vi "Shock.vi"() -> ()   [LabVIEW 2012]
uses:
  <vilib>/Instr/_visa.llb/Select Event Type.ctl
  <instrlib>/niHWS/nihws.llb/niHWS Open File Permissions ID.ctl
  <vilib>/DAQmx/write.llb/DAQmx Write (Digital Bool 1Line 1Point).vi
  <instrlib>/niHWS/nihws.llb/niHWS Write Analog WDT.vi
  <vilib>/DAQmx/miscellaneous.llb/DAQmx Fill In Error Info.vi
  <vilib>/express/express arith-compare/Formula/XNode/ExpressFormulaBlockNode.xnode
  <vilib>/ptbypt/NI_PtbyPt.lvlib
panel:
  out "Shock Countdown":dbl
  in  "Random":bool
  in  "shock time (ms)":u32
  in  "Shock Button":bool
  out "Shock":bool
  out "Click Value":i8
  out "Speed History":dbl(graph)
  in  "stop":bool
  out "Rec Time":dbl format="%#_3g"
  in  "Rec":bool
  in  "Path":path
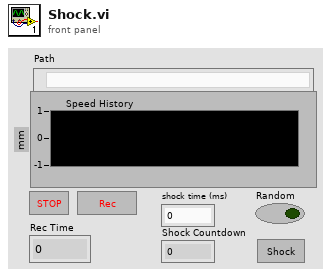
[diagram p1: front panel]
types:
  T1 = typedef "niHWS Open File Permissions ID.ctl" = enum32{"Read Only", "Read/Write Existing", "Read/Write/Create New", "Read/Write/Create New Always"}
  T2 = typedef "Select Event Type.ctl" = u32
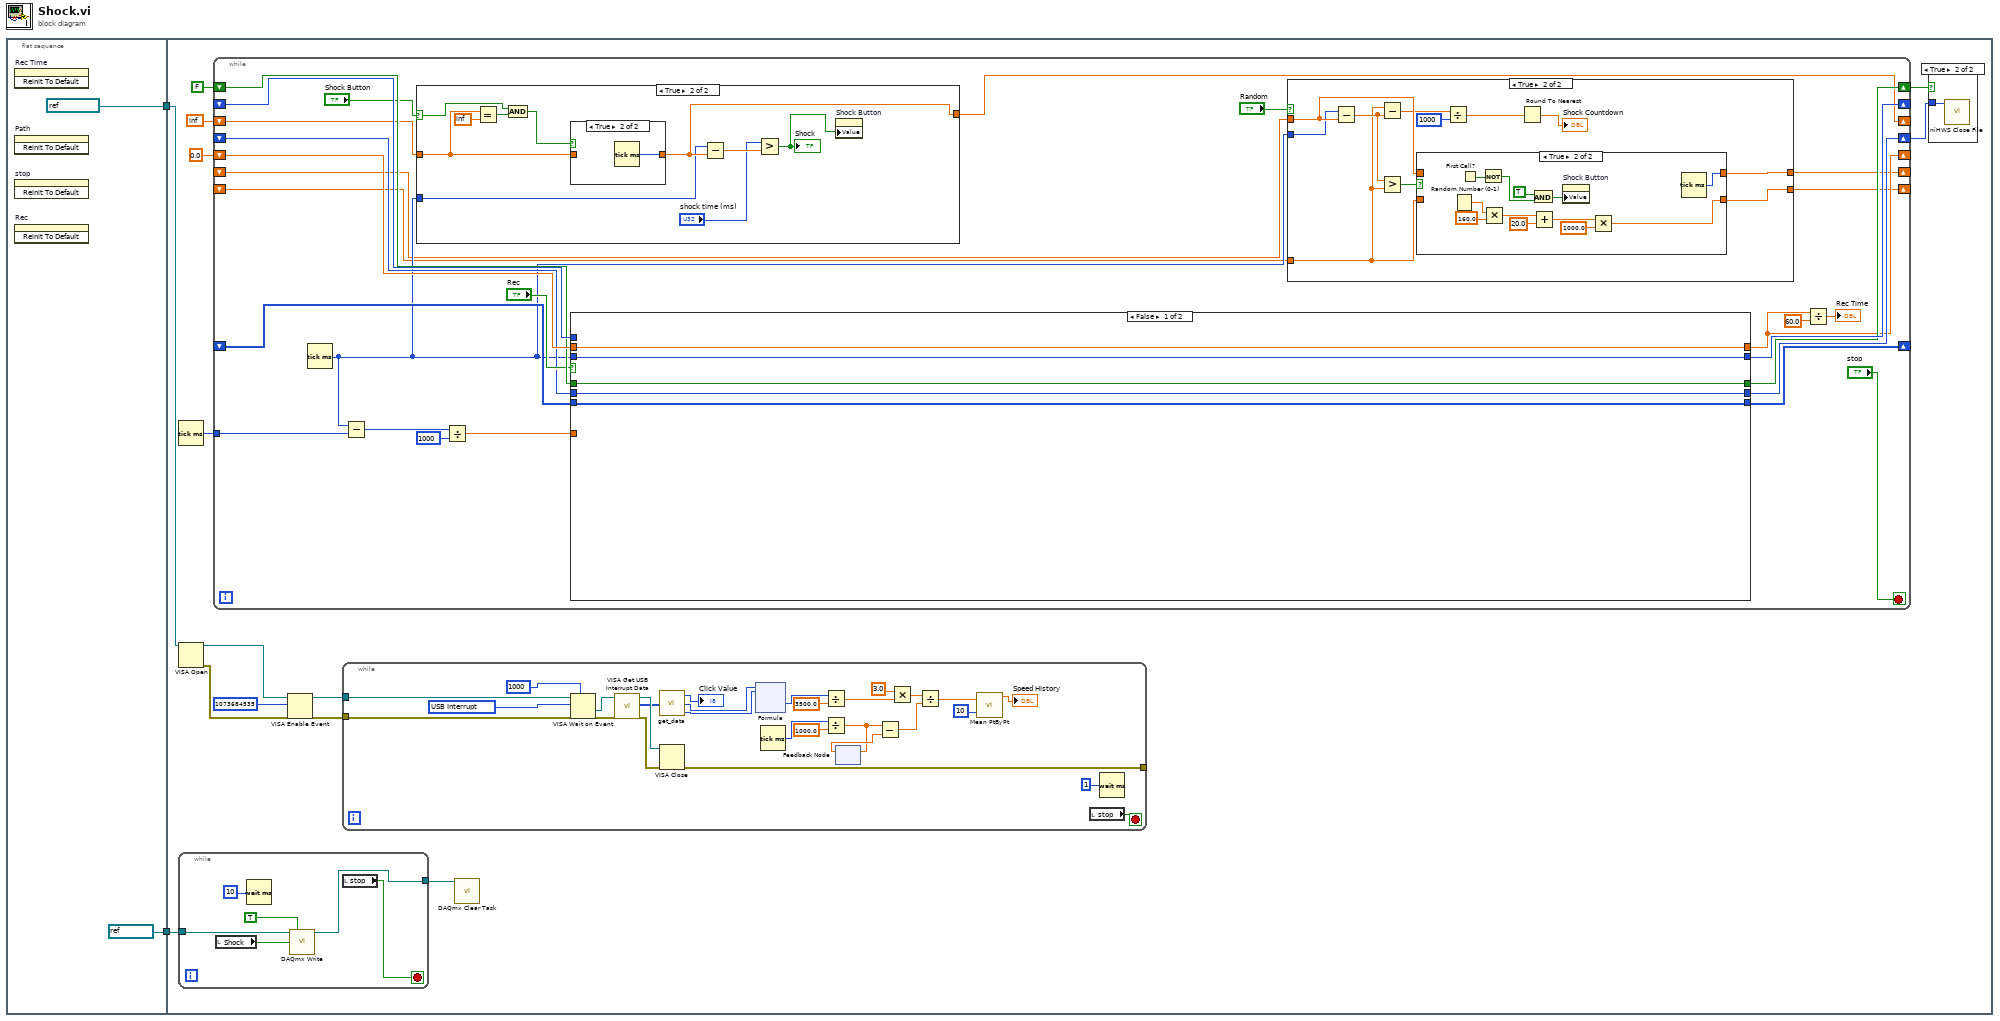
[diagram p0: block diagram]
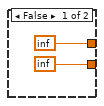
[diagram p3: hidden frame]
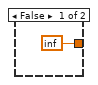
[diagram p5: hidden frame]
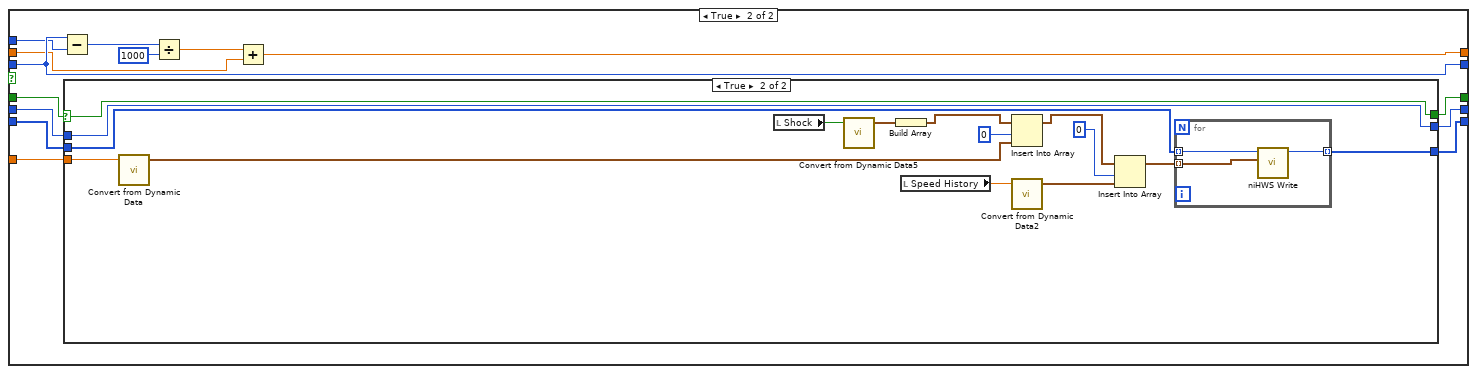
[diagram p7: hidden frame]
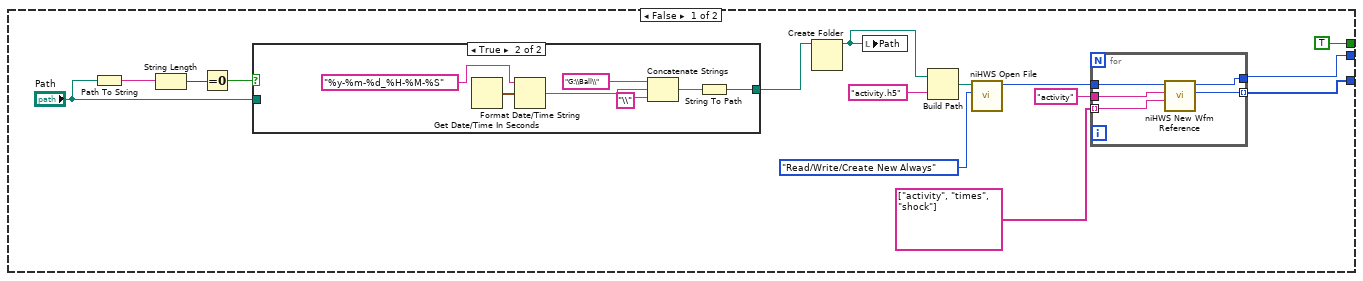
[diagram p8: hidden frame]
diagram:
  n1 = flat-sequence {
    tunnel: [refnum<visa-resource-name> "Mouse2" ("VISA resource name")] -> w2
    tunnel: [refnum<k21> "Shock" ("task/channels in")] -> w1
    tunnel: w2 -> [w8]
    tunnel: w1 -> [w7]
    frame #0 {
      n2 = invoke on="Rec Time" class="DigNum (strict)" method="Reinit To Default"() -> ()  [unwired: 3 in, 3 out]
      n3 = invoke on="Path" class="Path" method="Reinit To Default"() -> ()  [unwired: 3 in, 3 out]
      n4 = invoke on="stop" class="Bool (strict)" method="Reinit To Default"() -> ()  [unwired: 3 in, 3 out]
      n5 = invoke on="Rec" class="Bool (strict)" method="Reinit To Default"() -> ()  [unwired: 3 in, 3 out]
    }
    frame #1 {
      n6 = Tick Count (ms)() -> (millisecond timer value=w17:u32)
      n7 = VISA Open(VISA resource name=w8) -> (VISA resource name=w11:refnum<visa-resource-name>, error out=w10:errorcluster)  [unwired: 1 in, 3 out]
      n8 = while {
        tunnel: w7 -> [w60]
        tunnel: [w59] -> w6
        stop <- w62 stop-if-true
        n9 = local read "Shock"() -> (w57:bool)
        n10 = Wait (ms)(milliseconds to wait=u32 10) -> ()  [unwired: 1 out]
        n11 = call-poly <vilib>:"DAQmx Write.vi"("task/channels in"=w60, "auto start"=TRUE, "data"=w57) -> ("task out"=w59:refnum<k21>)  [unwired: 10 in, 2 out]
        n12 = local read "stop"() -> (w62:bool)
      }
      n13 = while {
        tunnel: w17 -> [w90]
        shift-right: [w89] -> _
        shift-left: _ -> [w88]
        shift-right: [w75] -> _
        shift-left: 0.0 -> [w87]
        shift-right: [w81] -> w15
        shift-left: FALSE -> [w82]
        shift-right: [w78] -> _
        shift-left: _ -> [w77]
        shift-right: [w79] -> w14
        shift-left: _ -> [w76]
        shift-right: [w71] -> _
        shift-left: inf -> [w70]
        shift-right: [w68] -> _
        shift-left: _ -> [w66]
        shift-right: [w65] -> _
        shift-left: _ -> [w64]
        stop <- "stop" stop-if-true
        n14 = Tick Count (ms)() -> (millisecond timer value=w67:u32)
        n15 = Subtract(x=w67, y=w90) -> (x-y=w85:u32)
        n16 = case shown="True" "Shock Button" {
          selector: "Shock Button" -> [_ w121]
          tunnel: w67 -> [_ w127]
          tunnel: [inf w128] -> w71
          tunnel: w70 -> [_ w123]
          frame False {
          }
          frame True {
            n17 = Equal?(x=w123, y=inf) -> (x = y?=w122:bool)
            n18 = And(x=w121, y=w122) -> (x .and. y?=w120:bool)
            n19 = case shown="True" w120 {
              tunnel: [w129 w130] -> w128
              tunnel: w123 -> [w129 _]
              frame False {
              }
              frame True {
                n20 = Tick Count (ms)() -> (millisecond timer value=w130:u32)
              }
            }
            n21 = Subtract(x=w127, y=w128) -> (x-y=w126:dbl)
            n22 = Greater?(x="shock time (ms)", y=w126) -> (0:w119:bool)
            "Shock" <- w119
            n23 = property on="Shock Button" class="Bool (strict)"("Value"=w119) -> ()  [unwired: 2 in, 2 out]
          }
        }
        n24 = Divide(x=w85, y=1000) -> (x/y=w83:dbl)
        n25 = case shown="False" "Rec" {
          tunnel: [w134 w146] -> w75
          tunnel: w83 -> [_ w140]
          tunnel: [w135 w149] -> w89
          tunnel: w67 -> [w135 w149]
          tunnel: w88 -> [_ w148]
          tunnel: w87 -> [w134 w147]
          tunnel: w82 -> [w133 w142]
          tunnel: [w133 w141] -> w81
          tunnel: [w131 w139] -> w79
          tunnel: [w132 w138] -> w78
          tunnel: w77 -> [w132 w137]
          tunnel: w76 -> [w131 w136]
          frame False {
          }
          frame True {
            n26 = Subtract(x=w149, y=w148) -> (x-y=w145:u32)
            n27 = case shown="True" w142 {
              selector: w142 -> [_ w192]
              tunnel: [TRUE w192] -> w141
              tunnel: w140 -> [_ w189]
              tunnel: [w152 w191] -> w139
              tunnel: [w151 w181] -> w138
              tunnel: w137 -> [_ w182]
              tunnel: w136 -> [_ w191]
              frame False {
                n28 = Path To String(path="Path") -> (string=w162:string)
                n29 = String Length(string=w162) -> (length=w163:i32)
                n30 = Equal To 0?(x=w163) -> (x = 0?=w158:bool)
                n31 = case shown="True" w158 {
                  tunnel: [w170 w171] -> w156
                  tunnel: "Path" -> [w170 _]
                  frame False {
                  }
                  frame True {
                    n32 = Get Date/Time In Seconds() -> (seconds since 1Jan1904=w177:timestamp)
                    n33 = Format Date/Time String(time format string (%c)="%y-%m-%d_%H-%M-%S", seconds (now)=w177) -> (date/time string=w174:string)  [unwired: 1 in]
                    n34 = Concatenate Strings("G:\\Ball\\", w174, "\\" ("string")) -> (w172:string)
                    n35 = String To Path(string=w172) -> (path=w171:path)
                  }
                }
                n36 = Create Folder(path (use dialog)=w156) -> (created path=w155:path)  [unwired: 2 in, 2 out]
                n37 = local write "Path"(w155) -> ()
                n38 = Build Path(base path=w155, name or relative path="activity.h5" ("search string")) -> (appended path=w159:path)
                n39 = call <instrlib>:"niHWS Open File.vi"("permissions (0:read only)"=niHWS_Open_File_Permissions_ID."Read/Write/Create New Always", "file path"=w159) -> ("file handle"=w150:u32)  [unwired: 8 in, 1 out]
                n40 = for {
                  tunnel: w150 -> [w169]
                  tunnel: [w168] -> w151 mode=indexing
                  tunnel: "activity" ("group name (empty)") -> [w167]
                  tunnel: string[] ["activity", "times", "shock"] -> [w166] mode=indexing
                  tunnel: [w165] -> w152
                  n41 = call <instrlib>:"niHWS New Wfm Reference.vi"("waveform name (empty)"=w166, "group name (empty)"=w167, "file handle in"=w169) -> ("waveform reference"=w168:u32, "file handle out"=w165:u32)  [unwired: 6 in, 1 out]
                }
              }
              frame True {
                n42 = call "Convert from Dynamic Data"("Dynamic Data Type"=w189) -> ("Waveform"=w188:waveform(dbl))  [unwired: 3 in]
                n43 = local read "Shock"() -> (w179:bool)
                n44 = call "Convert from Dynamic Data5"("Dynamic Data Type"=w179) -> ("Waveform"=w180:waveform(dbl))  [unwired: 3 in]
                n45 = Build Array(w180) -> (w178:waveform(dbl)[])
                n46 = local read "Speed History"() -> (w185:dbl)
                n47 = Insert Into Array(array=w178, index=0, new element=w188) -> (w186:waveform(dbl)[])
                n48 = call "Convert from Dynamic Data2"("Dynamic Data Type"=w185) -> ("Waveform"=w184:waveform(dbl))  [unwired: 3 in]
                n49 = Insert Into Array(array=w186, index=0, new element=w184) -> (w183:waveform(dbl)[])
                n50 = for {
                  tunnel: w182 -> [w195] mode=indexing
                  tunnel: w183 -> [w194] mode=indexing
                  tunnel: [w193] -> w181 mode=indexing
                  n51 = call-poly <instrlib>:"niHWS Write.vi"("analog waveform"=w194, "waveform reference in"=w195) -> ("waveform reference out"=w193:u32)  [unwired: 8 in, 1 out]
                }
              }
            }
            n52 = Divide(x=w145, y=1000) -> (x/y=w143:dbl)
            n53 = Add(x=w143, y=w147) -> (x+y=w146:dbl)
          }
        }
        n54 = case shown="True" "Random" {
          tunnel: [inf w103] -> w68
          tunnel: w67 -> [_ w101]
          tunnel: w66 -> [_ w102]
          tunnel: [inf w99] -> w65
          tunnel: w64 -> [_ w97]
          frame False {
          }
          frame True {
            n55 = Subtract(x=w101, y=w102) -> (x-y=w98:dbl)
            n56 = Subtract(x=w97, y=w98) -> (x-y=w96:dbl)
            n57 = Greater?(x=w98, y=w97) -> (0:w100:bool)
            n58 = case shown="True" w100 {
              tunnel: [w105 w113] -> w103
              tunnel: [w104 w111] -> w99
              tunnel: w102 -> [w105 _]
              tunnel: w97 -> [w104 _]
              frame False {
              }
              frame True {
                n59 = Random Number (0-1)() -> (number: 0 to 1=w117:dbl)
                n60 = First Call?() -> (First Call?: T/F=w110:bool)
                n61 = Not(x=w110) -> (.not. x?=w108:bool)
                n62 = Multiply(x=w117, y=160.0) -> (x*y=w114:dbl)
                n63 = And(x=TRUE ("Shock Button"), y=w108) -> (x .and. y?=w107:bool)
                n64 = Add(x=w114, y=20.0) -> (x+y=w112:dbl)
                n65 = property on="Shock Button" class="Bool (strict)"("Value"=w107) -> ()  [unwired: 2 in, 2 out]
                n66 = Multiply(x=w112, y=1000.0) -> (x*y=w111:dbl)
                n67 = Tick Count (ms)() -> (millisecond timer value=w113:u32)
              }
            }
            n68 = Divide(x=w96, y=1000) -> (x/y=w95:dbl)
            n69 = Round To Nearest(number=w95) -> (nearest integer value=→"Shock Countdown":dbl)
          }
        }
        n70 = Divide(x=w75, y=60.0) -> (x/y=→"Rec Time":dbl)
      }
      n71 = VISA Enable Event(8:w10, 10:u32 1073684535 ("event type"), 11:w11) -> (0:w13:errorcluster, 3:w12:refnum<visa-resource-name>)  [unwired: 1 out]
      n72 = while {
        tunnel: w12 -> [w46]
        tunnel: [w45] -> _
        tunnel: w13 -> [w38]
        stop <- w39 stop-if-true
        w37 = T2 1073684535 items=["Service Request"=1073684491, "Trigger"=3221168138, "Clear"=1073684493, "VXI Signal"=1073684512, "VXI/VME Interrupt"=3221168161, "VXI/VME Sysfail"=1073684509, "VXI/VME Sysreset"=1073684510, "GPIB CIC"=1073684498, "GPIB Talk"=1073684499, "GPIB Listen"=1073684500, "PXI Interrupt"=1073684514, "Serial Break"=1073684515, "Serial TermChar"=1073684516, "Serial CTS"=1073684521, "Serial DSR"=1073684522, "Serial DCD"=1073684524, "Serial RI"=1073684526, "Serial Character"=1073684533, "USB Interrupt"=1073684535, "All Enabled"=1073709055] ("Event Type")
        n73 = VISA Wait on Event(7:u32 1000 ("timeout (0)"), 8:w38, 10:w37, 11:w46) -> (0:w42:errorcluster, 1:w41:refnum<visa-resource-name>)  [unwired: 3 out]
        n74 = call <vilib>:"VISA Get USB Interrupt Data.vi"("error in (no error)"=w42, "VISA USB Intr Event"=w41) -> ("error out"=w44:errorcluster, "data buffer"=w35:u8[], "VISA USB Intr Event out"=w43:refnum<visa-resource-name>)  [unwired: 7 out]
        n75 = call "get_data.vi"("data buffer"=w35) -> ("Click Value"=→"Click Value":i8, "X Value"=w19:i8, "Y Value"=w20:i8)
        n76 = VISA Close(VISA resource name=w43, error in (no error)=w44) -> (error out=w45:errorcluster)
        n77 = xnode ("Formula")("X1"=w19, "X2"=w20) -> ("Result"=w32:i8)  [unwired: 1 in, 1 out]
        n78 = Tick Count (ms)() -> (millisecond timer value=w30:u32)
        n79 = Divide(x=w32, y=3500.0 ("DPI")) -> (x/y=w27:dbl)
        n80 = Divide(x=w30, y=1000.0) -> (x/y=w28:dbl)
        n81 = feedback #1() -> (w33:dbl)  [unwired: 1 in]
        n82 = feedback-in #1(w28) -> ()
        n83 = Subtract(x=w28, y=w33) -> (x-y=w31:dbl)
        n84 = Multiply(x=3.0, y=w27) -> (x*y=w26:dbl)
        n85 = Divide(x=w26, y=w31) -> (x/y=w23:dbl)
        n86 = call <vilib>:"Mean PtByPt.vi"("x"=w23, "sample length"=10) -> ("mean"=→"Speed History":dbl)  [unwired: 2 in, 1 out]
        n87 = local read "stop"() -> (w39:bool)
        n88 = Wait (ms)(milliseconds to wait=u32 1) -> ()  [unwired: 1 out]
      }
      n89 = call <vilib>:"DAQmx Clear Task.vi"("task in"=w6) -> ()  [unwired: 14 in, 1 out]
      n90 = case shown="True" w15 {
        tunnel: w14 -> [_ w63]
        frame False {
        }
        frame True {
          n91 = call <instrlib>:"niHWS Close File.vi"("file handle"=w63) -> ()  [unwired: 10 in, 1 out]
        }
      }
    }
  }
